vi "verfluchter_Kackdreck.vi"(7 "XAS (false, def), XPS (true)":bool, 9 "Last Motor moved in Scan":u16(ring) items=["none", "1", "2", "3", "4", "all"]) -> (1 "Last Motor Moved in Scan (Out)":u16(ring) items=["none", "1", "2", "3", "4", "all"])   [LabVIEW 2018]
uses:
  Global_Next_Scan_Position.vi
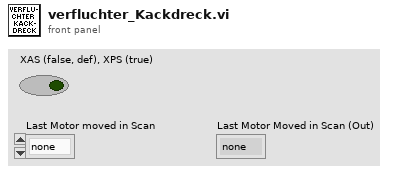
[diagram p1: front panel]
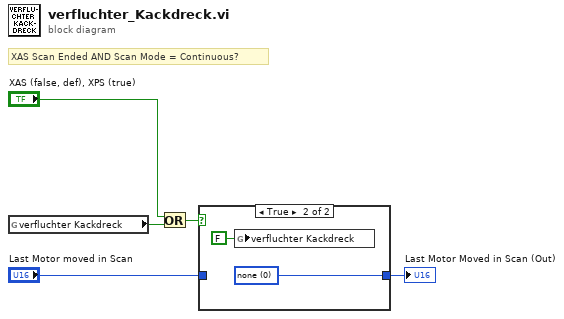
[diagram p0: block diagram]
diagram:
  # "XAS Scan Ended AND Scan Mode = Continuous?"
  n1 = global read "Global_Next_Scan_Position.vi" "verfluchter Kackdreck"() -> (w3:bool)
  n2 = Or(x="XAS (false, def), XPS (true)", y=w3) -> (x .or. y?=w1:bool)
  n3 = case shown="True" w1 {
    tunnel: "Last Motor moved in Scan" -> [w6 _]
    tunnel: [w6 w8] -> w4
    frame False {
    }
    frame True {
      w8 = u16 0 items=["none", "1", "2", "3", "4", "all"] ("Last Motor Moved in Scan (Out) 2")
      n4 = global write "Global_Next_Scan_Position.vi" "verfluchter Kackdreck"(FALSE ("verfluchter Kackdreck")) -> ()
    }
  }
  "Last Motor Moved in Scan (Out)" <- w4
